vi "KB-内环计算拐点的最高值.vi"(11 "二维内环数组":dbl[][](array[numeric])=array101x102[10302 elements]) -> (3 "结果":dbl[](array[numeric]))   [LabVIEW 2015]
uses:
  <vilib>/Math Plots/3D Math Plots/3D Surface/3D Surface XCtrl/3D Surface.xctl
  <vilib>/Math Plots/3D Math Plots/3D Surface/3D Surface Datatype/Public/Plot Helper (Matrix).vi
  <vilib>/Math Plots/3D Math Plots/3D Surface/3D Surface Datatype/3D Surface Datatype.lvclass
  <vilib>/Analysis/NI_AAL_SigProc.lvlib
panel:
  out "index  2":i32
  out "index":i32
  out "波形图 5":dbl[](graph)
  out "Locations":dbl[](array[numeric]) caption="位置"
  out "波形图 2":dbl[](graph)
  out "大小":i32[](array[numeric])
  out "内外环":refnum<class "3D Plot Datatype.lvclass">[](xcontrol) caption="0.38"
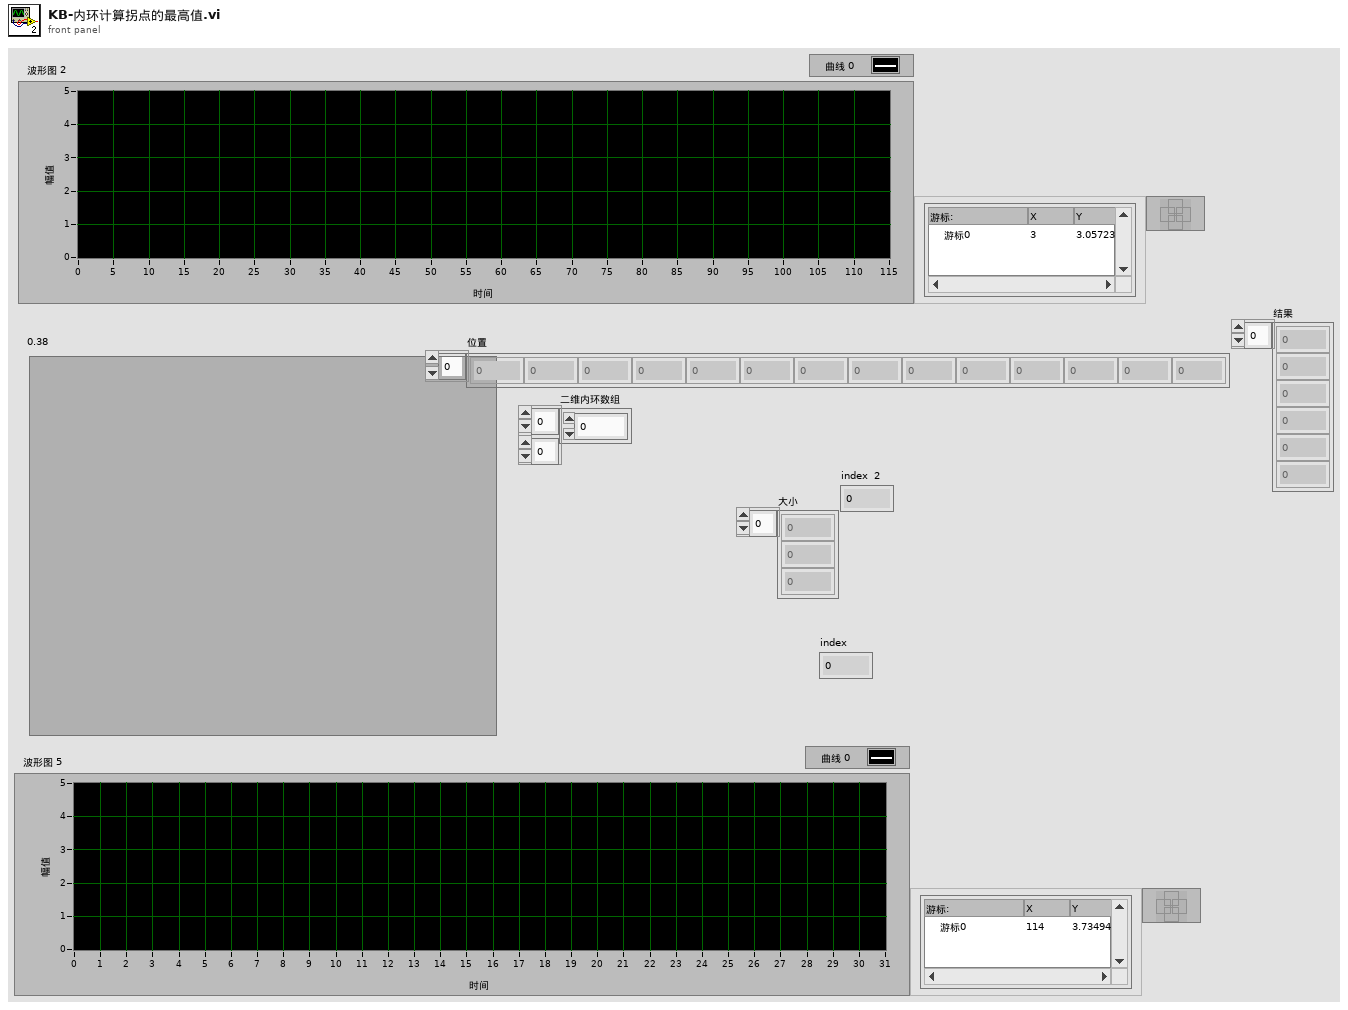
[diagram p1: front panel]
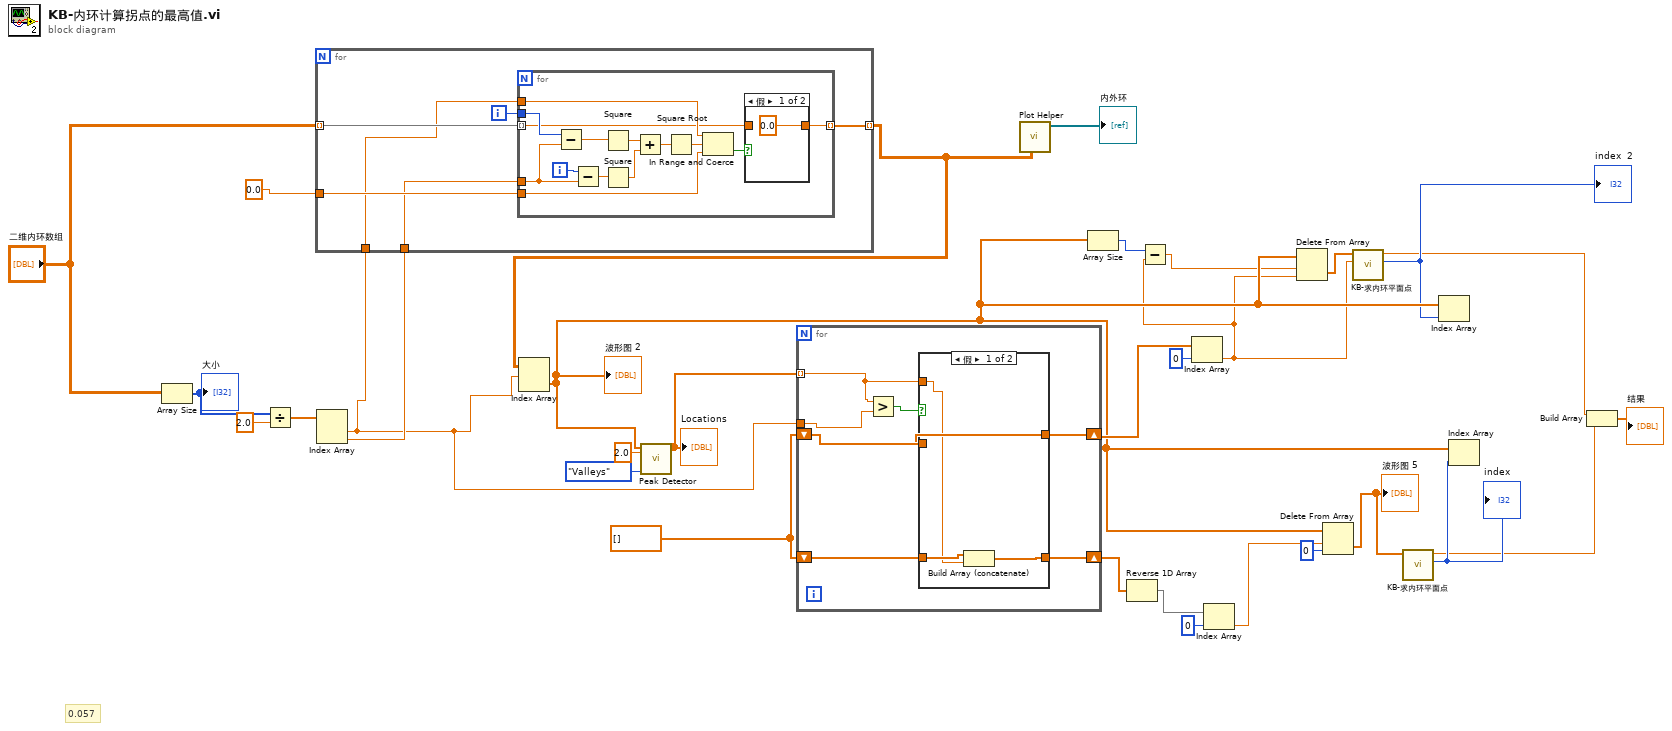
[diagram p0: block diagram]
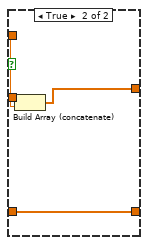
[diagram p2: hidden frame]
diagram:
  w22 = dbl[] []
  # "0.057"
  n1 = Array Size(array="二维内环数组") -> (size(s)=w29:i32[])
  "大小" <- w29
  n2 = Divide(x=w29, y=2.0) -> (x/y=w28:dbl[])
  n3 = Index Array(array=w28) -> (element #1=w15:dbl, element #2=w24:dbl)  [unwired: 2 in]
  n4 = for {
    tunnel: "二维内环数组" -> [w35] mode=indexing
    tunnel: 0.0 ("y") -> [w36]
    tunnel: [w34] -> w16 mode=indexing
    tunnel: w15 -> [w33]
    tunnel: w24 -> [w32]
    i -> [w37]
    n5 = for {
      tunnel: w37 -> [w51]
      tunnel: w32 -> [w48]
      tunnel: w33 -> [w42]
      tunnel: w36 -> [w41]
      tunnel: w35 -> [w39] mode=indexing
      tunnel: [w38] -> w34 mode=indexing
      i -> [w49]
      n6 = Subtract(x=w51, y=w48) -> (x-y=w50:dbl)
      n7 = Subtract(x=w49, y=w48) -> (x-y=w47:dbl)
      n8 = Square(x=w50) -> (x^2=w45:dbl)
      n9 = Square(x=w47) -> (x^2=w46:dbl)
      n10 = Add(x=w45, y=w46) -> (x+y=w44:dbl)
      n11 = Square Root(x=w44) -> (sqrt(x)=w43:dbl)
      n12 = In Range and Coerce(upper limit=w42, x=w43, lower limit=w41) -> (In Range?=w40:bool)  [unwired: 1 out]
      n13 = case shown="假" w40 {
        tunnel: w39 -> [_ w53]
        tunnel: [0.0 w53] -> w38
        frame False {
        }
        frame True {
        }
      }
    }
  }
  n14 = Index Array(array=w16, index (row)=w15) -> (element=w11:dbl[])  [unwired: 1 in]
  "波形图 2" <- w11
  n15 = call <vilib>:"Peak Detector.vi"("peaks/valleys"=enum32{"Peaks", "Valleys"}."Valleys", "threshold"=2.0, "X"=w11) -> ("Locations"=w23:dbl[])  [unwired: 4 in, 4 out]
  "Locations" <- w23
  n16 = for {
    tunnel: w23 -> [w58] mode=indexing
    shift-right: [w59] -> w17
    shift-left: w22 -> [w60]
    tunnel: w15 -> [w56]
    shift-right: [w54] -> w21
    shift-left: w22 -> [w55]
    n17 = Greater?(x=w58, y=w56) -> (0:w57:bool)
    n18 = case shown="假" w57 {
      tunnel: w60 -> [w64 w68]
      tunnel: w58 -> [w62 w67]
      tunnel: [w64 w66] -> w59
      tunnel: w55 -> [w63 w65]
      tunnel: [w61 w65] -> w54
      frame False {
        n19 = Build Array (concatenate)(w63, w62) -> (w61:dbl[])
      }
      frame True {
        n20 = Build Array (concatenate)(w68, w67) -> (w66:dbl[])
      }
    }
  }
  n21 = call-poly <vilib>:"Plot Helper.vi"("z matrix"=w16) -> ("3D Plot lvclass Array out"=→"内外环":refnum<class "3D Plot Datatype.lvclass">[])  [unwired: 5 in, 5 out]
  n22 = Array Size(array=w11) -> (size(s)=w12:i32)
  n23 = Reverse 1D Array(array=w21) -> (reversed array=w20:dbl[])
  n24 = Index Array(array=w17, index=0 ("索引")) -> (element=w9:dbl)
  n25 = Subtract(x=w12, y=w9) -> (x-y=w10:dbl)
  n26 = Index Array(array=w20, index=0 ("索引")) -> (element=w6:dbl)
  n27 = Delete From Array(array=w11, length=w10, index=w9) -> (deleted portion=w8:dbl[])  [unwired: 1 out]
  n28 = Delete From Array(array=w11, length=w6, index=0 ("索引")) -> (deleted portion=w4:dbl[])  [unwired: 1 out]
  "波形图 5" <- w4
  n29 = call "KB-求内环平面点.vi"("offset"=w9, "波形图 7"=w8) -> ("index"=w7:i32, "元素"=w2:dbl)  [unwired: 8 in]
  "index  2" <- w7
  n30 = call "KB-求内环平面点.vi"("波形图 7"=w4) -> ("index"=w3:i32, "元素"=w1:dbl)  [unwired: 9 in]
  "index" <- w3
  n31 = Index Array(array=w11, index=w7) -> ()  [unwired: 1 out]
  n32 = Index Array(array=w11, index=w3) -> ()  [unwired: 1 out]
  n33 = Build Array(w2, w1) -> (→"结果":dbl[])
